vi "Configure Multi Eval Meas Spectrum ACLR Adjacent Channel Enabled.vi"(6 "NR (On)":bool=TRUE, 7 "UTRA 2 (On)":bool=TRUE, 8 "error in (no error)":errorcluster, 9 "UTRA 1 (On)":bool=TRUE, 10 "Instance (1)":T1=1, 11 "VISA resource name":refnum<visa-resource-name>) -> (0 "error out":errorcluster, 3 "VISA resource name out":refnum<visa-resource-name>)   [LabVIEW 2020, in "Rohde&Schwarz CMWXP NR FR1 Measurement.lvlib"]
doc: "Enables or disables the evaluation of the first adjacent UTRA channels, second adjacent UTRA channels and first adjacent NR channels.\n\nAttribute:\nRSCMWXPNRFR1M_ATTR_MULTI_EVAL_MEAS_SPECTRUM_ACLR_ADJACENT_CHANNEL_ENABLED\n\nRemote-control command:\nCONFigure:NRSub:MEAS<i>:MEValuation:SPECtrum:ACLR:ENABle"
uses:
  <instrlib>/Rohde&Schwarz CMWXP NR FR1 Measurement/Rohde&Schwarz CMWXP NR FR1 Measurement.lvlib
  <instrlib>/Rohde&Schwarz CMWXP NR FR1 Measurement/Private/_Instance.ctl
  <instrlib>/Rohde&Schwarz CMWXP NR FR1 Measurement/Private/rsidr_core.llb/rsidr_core.lvlib
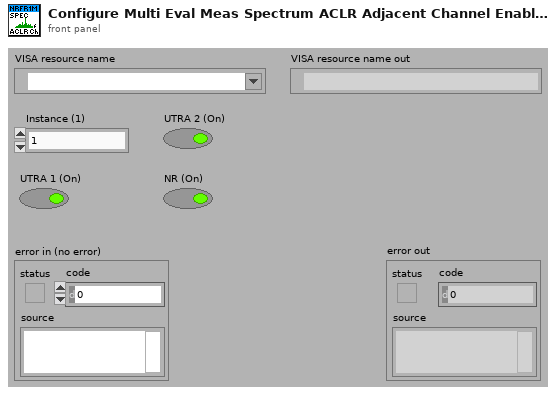
[diagram p1: front panel]
types:
  T1 = typedef "Rohde&Schwarz CMWXP NR FR1 Measurement.lvlib/_Instance.ctl" = i32
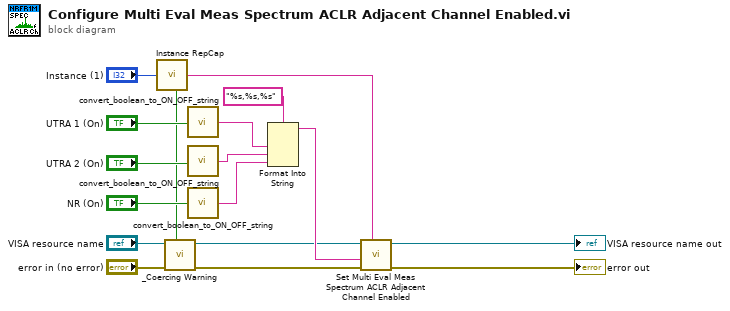
[diagram p0: block diagram]
diagram:
  n1 = call <instrlib>:"Instance RepCap.vi"("Instance In"="Instance (1)") -> ("In Range?"=w1:bool, "RepCap Identifier Out"=w16:string)  [unwired: 1 in]
  n2 = call <instrlib>:"_Coercing Warning.vi"("In Range?"=w1, "error in (no error)"="error in (no error)", "VISA resource name"="VISA resource name") -> ("error out"=w3:errorcluster, "VISA resource name out"=w2:refnum<visa-resource-name>)  [unwired: 7 in]
  n3 = call <instrlib>:"convert_boolean_to_ON_OFF_string.vi"("boolean value in"="UTRA 1 (On)") -> ("string value out"=w11:string)  [unwired: 4 in]
  n4 = call <instrlib>:"convert_boolean_to_ON_OFF_string.vi"("boolean value in"="UTRA 2 (On)") -> ("string value out"=w10:string)  [unwired: 4 in]
  n5 = call <instrlib>:"convert_boolean_to_ON_OFF_string.vi"("boolean value in"="NR (On)") -> ("string value out"=w9:string)  [unwired: 4 in]
  n6 = Format Into String(format string="%s,%s,%s", w11, w10, w9) -> (resulting string=w8:string)  [unwired: 2 in, 1 out]
  n7 = call "Set Multi Eval Meas Spectrum ACLR Adjacent Channel Enabled"("Repeated Capabilities"=w16, "error in (no error)"=w3, "Multi Eval Meas Spectrum ACLR Adjacent Channel Enabled ()"=w8, "instrument handle"=w2) -> ("error out"=→"error out":errorcluster, "instrument handle out"=→"VISA resource name out":refnum<visa-resource-name>)  [unwired: 6 in]
